vi "shutter.vi"(2 "error in (no error)":errorcluster, 3 "Boolean":bool, 4 "lines":tag="6052E/port0/line0") -> (0 "error out":errorcluster)   [LabVIEW 2015]
uses:
  <vilib>/DAQmx/write.llb/DAQmx Write (Digital Bool 1Line 1Point).vi
  <vilib>/DAQmx/create/channels.llb/DAQmx Create Channel (DO-Digital Output).vi
  <vilib>/DAQmx/miscellaneous.llb/DAQmx Fill In Error Info.vi
  <resource>/objmgr/daqmx.rc
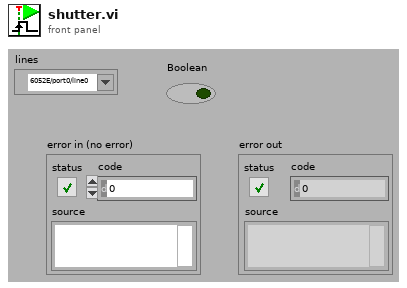
[diagram p1: front panel]
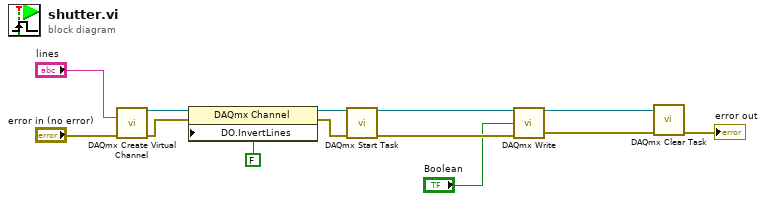
[diagram p0: block diagram]
diagram:
  n1 = call-poly <vilib>:"DAQmx Create Virtual Channel.vi"("lines"="lines", "error in"="error in (no error)") -> ("task out"=w8:refnum<k21>, "error out"=w6:errorcluster)  [unwired: 12 in]
  n2 = property class="DAQmx Channel"(reference=w8, error in=w6, "DO.InvertLines"=FALSE) -> (reference out=w7:refnum<k21>, error out=w5:errorcluster)
  n3 = call <vilib>:"DAQmx Start Task.vi"("task/channels in"=w7, "error in"=w5) -> ("task out"=w12:refnum<k21>, "error out"=w11:errorcluster)  [unwired: 12 in]
  n4 = call-poly <vilib>:"DAQmx Write.vi"("task/channels in"=w12, "data"="Boolean", "error in"=w11) -> ("task out"=w10:refnum<k21>, "error out"=w9:errorcluster)  [unwired: 10 in, 1 out]
  n5 = call <vilib>:"DAQmx Clear Task.vi"("task in"=w10, "error in"=w9) -> ("error out"=→"error out":errorcluster)  [unwired: 13 in]
